vi "VG_ST5520.vi"() -> ()   [LabVIEW 2020]
panel:
  in  "ST5520":string
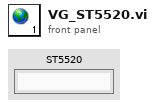
[diagram p1: front panel]
diagram:
